vi "MEScope_SpanCalOhms.vi"(8 "error in (no error)":errorcluster, 10 "nDelayValue":i32, 11 "nScale":i32) -> (0 "error out":errorcluster, 3 "Return Code":i32)   [LabVIEW 2015]
doc: "MEScope_SpanCalOhms \nDescription:\nThis function will read the ADC offset for Ohms, after first setting the hardware for the appropriate scale. The values are stored in the Local EEPROM structure.\nDetail:\nint MEScope_SpanCalOhms (\nint nScale, \nint nDelayValue\n);\n\nParameters:\nint nScale - which scale to use (M5_OHMS_40 to M5_OHMS_4MEG)\n\nint nDelayValue - A delay value in mS, based on the table below:\n\nScale 40 400 4 k 40 k 400 k 4 Meg\nDelay 100 100 100 500 2000 15000\n\n\nReturn Values:\nThis function returns a 0 if the function completed successfully. A non-zero return code will indicate error. \nRemarks:\nIn order to facilitate easier calibration on the WaveTek calibrator, call this function with the appropriate scale before selecting the ohms value on the Wavetek (in which case, the delay value can always be 0). Make a second call with the proper delay for the actual calibration process.\n\nScale definitions:\n#define M5_OHMS_40 0\n#define M5_OHMS_400 1\n#define M5_OHMS_4K 2\n#define M5_OHMS_40K 3\n#define M5_OHMS_400K 4\n#define M5_OHMS_4MEG 5\n\nSerial Command packet: \nn/a"
uses:
  ScannerDiagDLL.dll
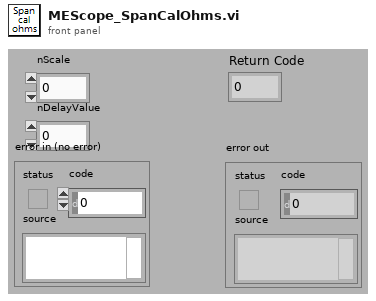
[diagram p1: front panel]
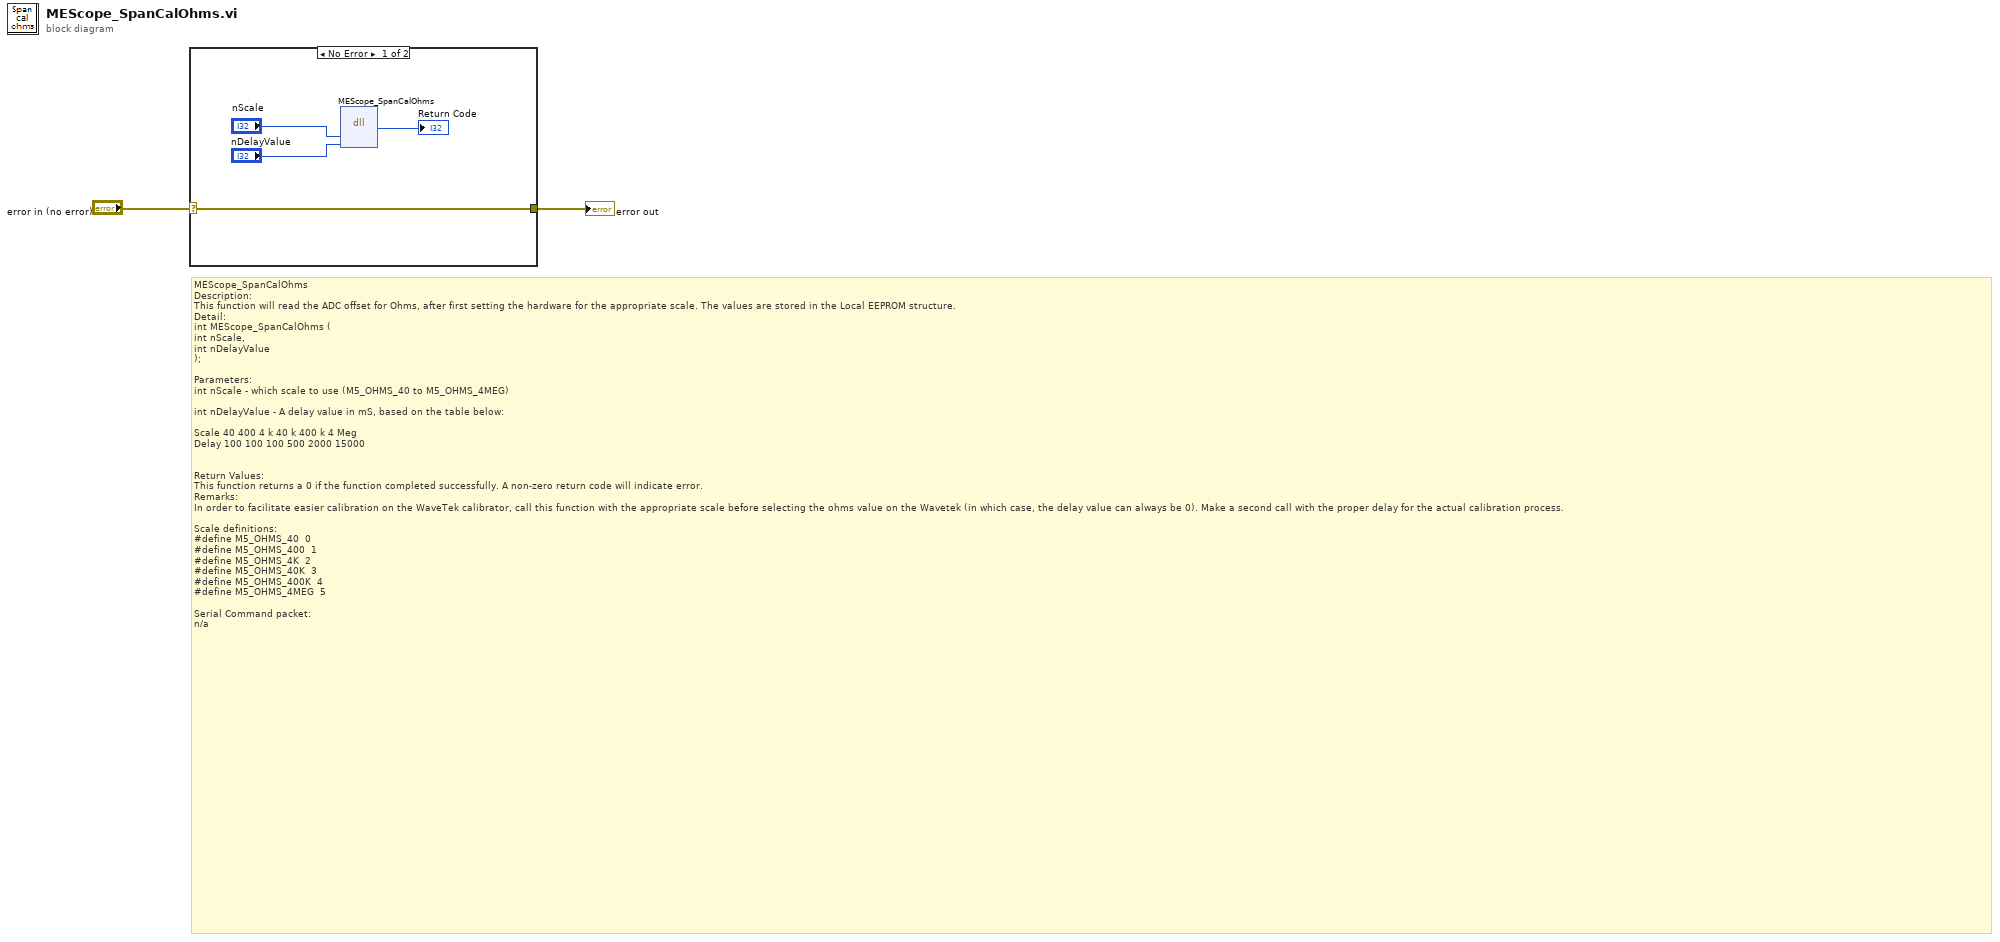
[diagram p0: block diagram]
diagram:
  # "MEScope_SpanCalOhms  \nDescription:\nThis function will read the ADC offset for Ohms, after first setting the hardware for the appropriate scale. The values are stored in the Local EEPROM structure.\nDetail:\nint MEScope_SpanCalOhms (\nint nScale, \nint nDelayValue\n);\n\nParameters:\nint nScale - which scale to use (M5_OHMS_40 to M5_OHMS_4MEG)\n\nint nDelayValue - A delay value in mS, based on the table below:\n\nScale\t40\t400\t4 k\t40 k\t400 k\t4 Meg\nDelay\t100\t100\t100\t500\t2000\t15000\n\n\nReturn Values:\nThis function returns a 0 if the function completed successfully. A non-zero return code will indicate error. \nRemarks:\nIn order to facilitate easier calibration on the WaveTek calibrator, call this function with the appropriate scale before selecting the ohms value on the Wavetek (in which case, the delay value can always be 0). Make a second call with the proper delay for the actual calibration process.\n\nScale definitions:\n#define M5_OHMS_40\t\t0\n#define M5_OHMS_400\t\t1\n#define M5_OHMS_4K\t\t2\n#define M5_OHMS_40K\t\t3\n#define M5_OHMS_400K\t\t4\n#define M5_OHMS_4MEG\t\t5\n\nSerial Command packet: \nn/a"
  n1 = case shown="No Error" "error in (no error)" {
    selector: "error in (no error)" -> [w5 w7]
    tunnel: [w5 w7] -> w1
    frame No Error {
      n2 = dll-call lib="C:/ModisEdge/TabletScope/Test Sequence/Code Modules/DLL/ScannerDiagDLL.dll" fn="MEScope_SpanCalOhms" ("TripoliDLL.dll:Test_WirelessLANPort")("nScale"="nScale", "nDelayValue"="nDelayValue") -> ("return type"=→"Return Code":i32)  [unwired: 5 in, 2 out]
    }
    frame Error {
    }
  }
  "error out" <- w1
